vi "Notifier.vi"() -> ()   [LabVIEW 2020]
panel:
  out "Numeric 2":dbl
  in  "Stop 3":bool
  in  "Stop 2":bool
  in  "Stop":bool
  in  "Generate":bool
  out "Numeric":dbl
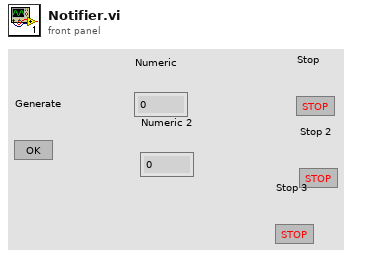
[diagram p1: front panel]
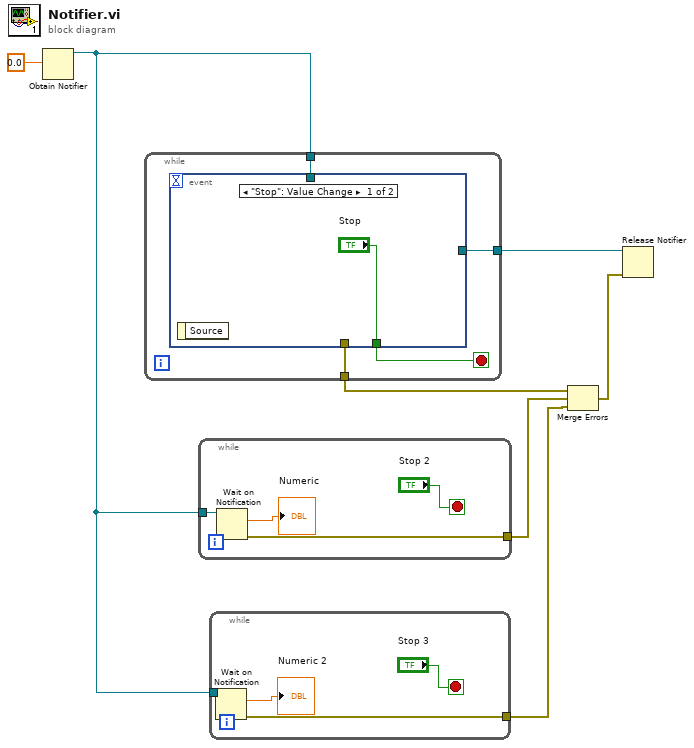
[diagram p0: block diagram]
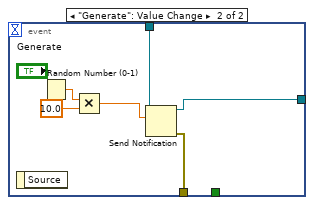
[diagram p2: hidden frame]
diagram:
  n1 = Obtain Notifier(notification data type=0.0) -> (notifier out=w1:refnum<notifier>)  [unwired: 3 in, 2 out]
  n2 = while {
    tunnel: w1 -> [w11]
    tunnel: [w10] -> w6
    tunnel: [w8] -> w4
    stop <- w9 stop-if-true
    n3 = event shown="[0] \"Stop\": Value Change" {
      selector: _ -> [_ _]
      dyn-events: _ -> [_ _]
      timeout: _ -> [_ _]
      tunnel: w11 -> [_ w15]
      tunnel: [_ w14] -> w10
      tunnel: ["Stop" _] -> w9
      tunnel: [_ w13] -> w8
      event "Stop": Value Change {
        n4 = event-data() -> ()  [unwired: 1 in, 1 out]
      }
      event "Generate": Value Change {
        n5 = event-data() -> ()  [unwired: 1 in, 1 out]
        n6 = Random Number (0-1)() -> (number: 0 to 1=w18:dbl)
        n7 = Multiply(x=w18, y=10.0) -> (x*y=w16:dbl)
        n8 = Send Notification(notification=w16, notifier=w15) -> (notifier out=w14:refnum<notifier>, error out=w13:errorcluster)  [unwired: 1 in]
      }
    }
  }
  n9 = while {
    tunnel: w1 -> [w22]
    tunnel: [w20] -> w5
    stop <- "Stop 2" stop-if-true
    n10 = Wait on Notification(notifier=w22) -> (notification=→"Numeric":dbl, error out=w20:errorcluster)  [unwired: 3 in, 2 out]
  }
  n11 = while {
    tunnel: w1 -> [w26]
    tunnel: [w24] -> w2
    stop <- "Stop 3" stop-if-true
    n12 = Wait on Notification(notifier=w26) -> (notification=→"Numeric 2":dbl, error out=w24:errorcluster)  [unwired: 3 in, 2 out]
  }
  n13 = Merge Errors "Merge Errors"(w4, w5, w2) -> (w3:errorcluster)
  n14 = Release Notifier(notifier=w6, error in (no error)=w3) -> ()  [unwired: 1 in, 3 out]
